vi "FightBot.vi"   [LabVIEW 2016, in "SumoRobot.lvrbt"]
uses:
  SumoRobot.lvrbt
  <vilib>/NXT/Block Support/NXT_OutputPort.ctl
  <vilib>/NXT/Block Support/NXT_InputPort.ctl
  <vilib>/NXT/Dual Mode Library/Sensors/Touch_Pressed.vi
  <vilib>/NXT/Dual Mode Library/Sensors/EV3_Color_Reflect.vi
  <vilib>/NXT/NXTIO Xnodes/NXTIONodeSubVIs/NXTMoveMotors.vi
  <vilib>/NXT/Dual Mode Library/Sensors/EV3_Ultrasonic_IN.vi
  <vilib>/NXT/Dual Mode Library/Display/drawNumber_float.vi
  <vilib>/NXT/Dual Mode Library/Display/drawText.vi
  <vilib>/NXT/Dual Mode Library/Sound/PlayRedPianoFile.vi
  <vilib>/NXT/Subs/LVHSConnector.ctl
  <vilib>/NXT/NXTIO Xnodes/AddressXNode/NXTIOAddress.xnode
  <vilib>/NXT/NXTIO Xnodes/NXTIOXNode/NXTIO.xnode
  <vilib>/NXT/LegoClasses/BrickReference/BrickReference.lvclass
types:
  T1 = typedef "NXT_InputPort.ctl" = u32
  T2 = typedef "NXT_OutputPort.ctl" = u8
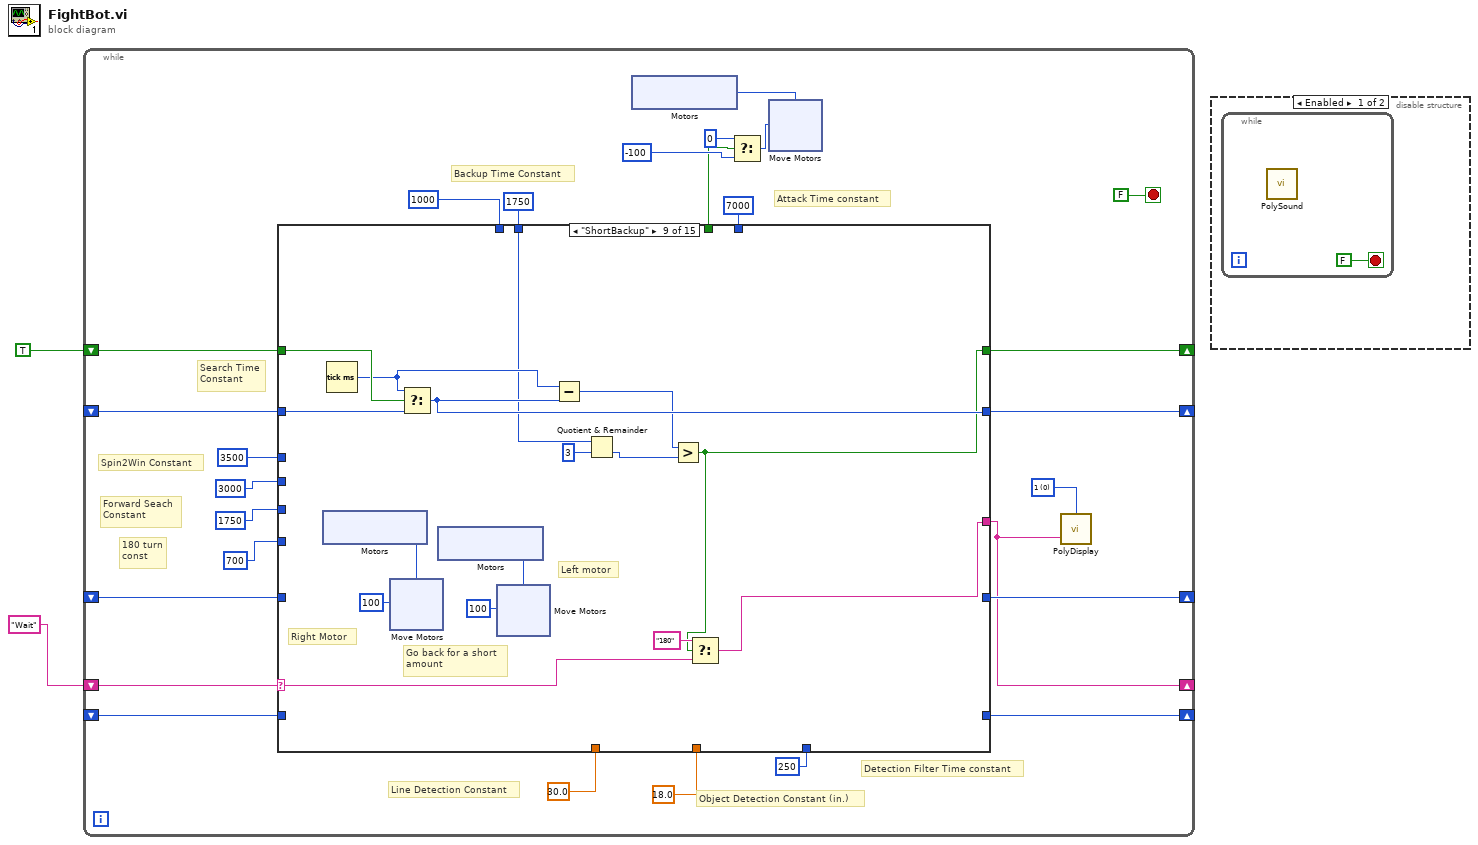
[diagram p0: block diagram]
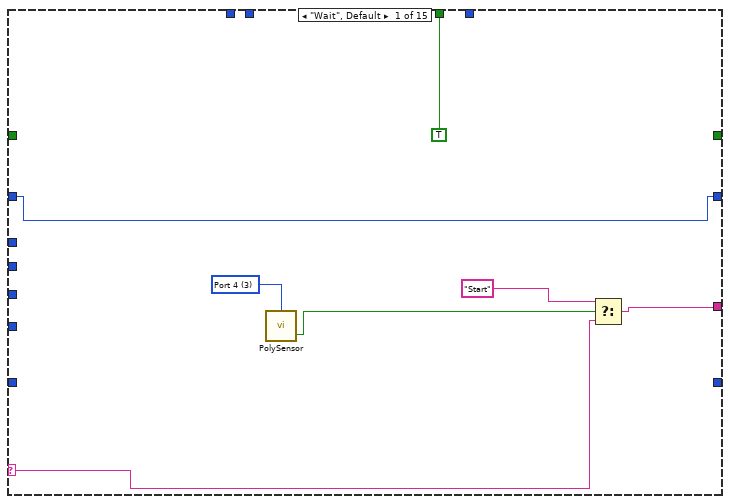
[diagram p3: hidden frame]
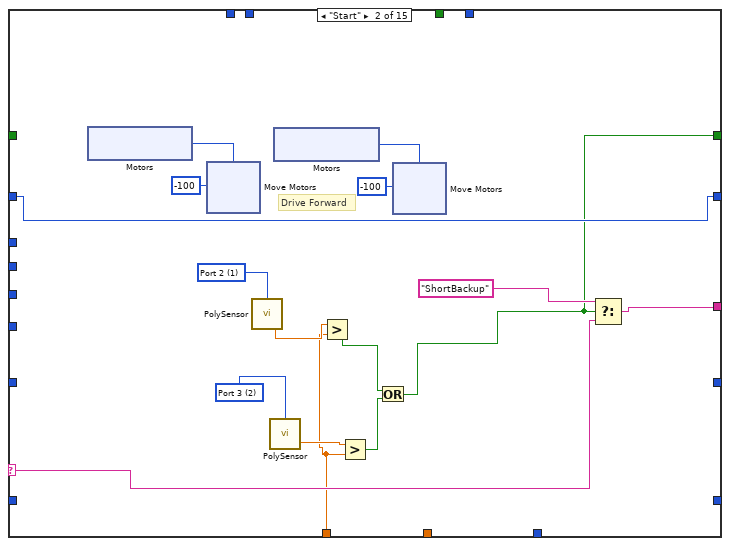
[diagram p4: hidden frame]
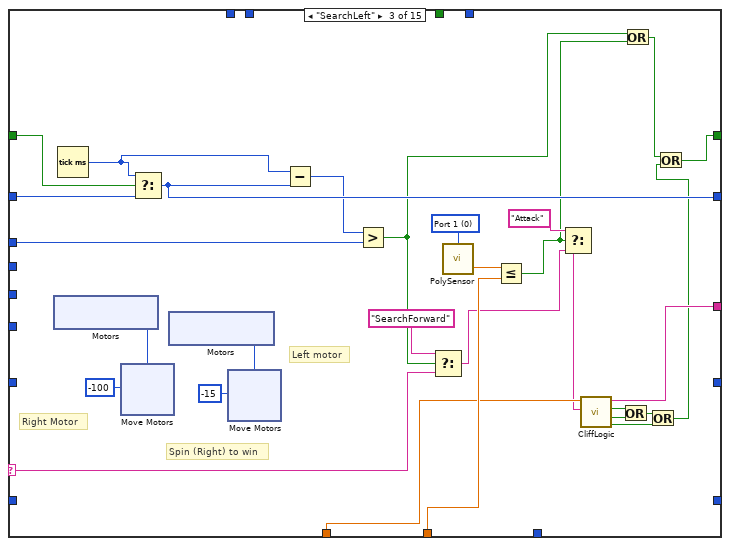
[diagram p5: hidden frame]
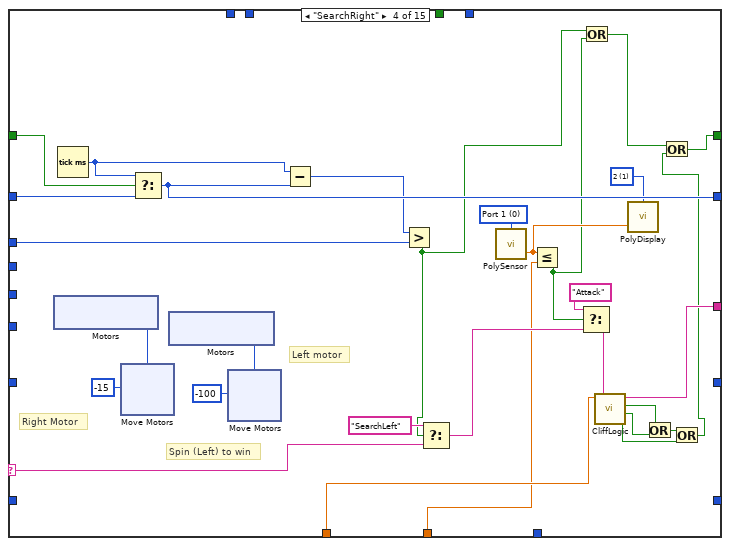
[diagram p6: hidden frame]
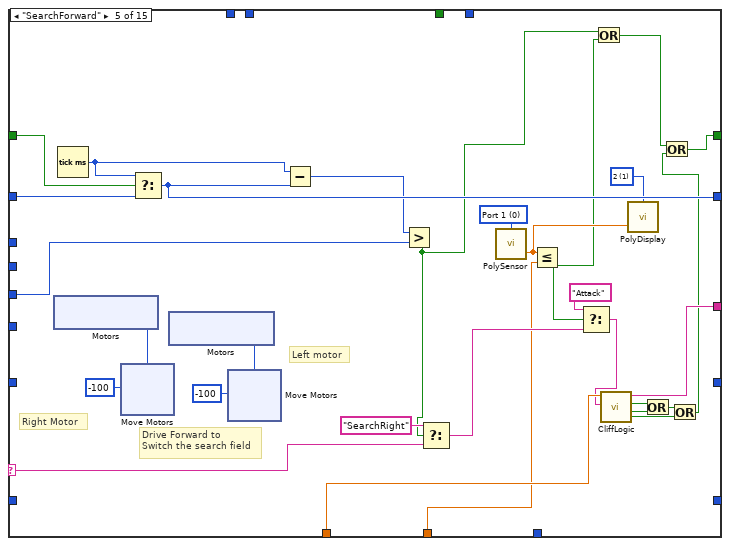
[diagram p7: hidden frame]
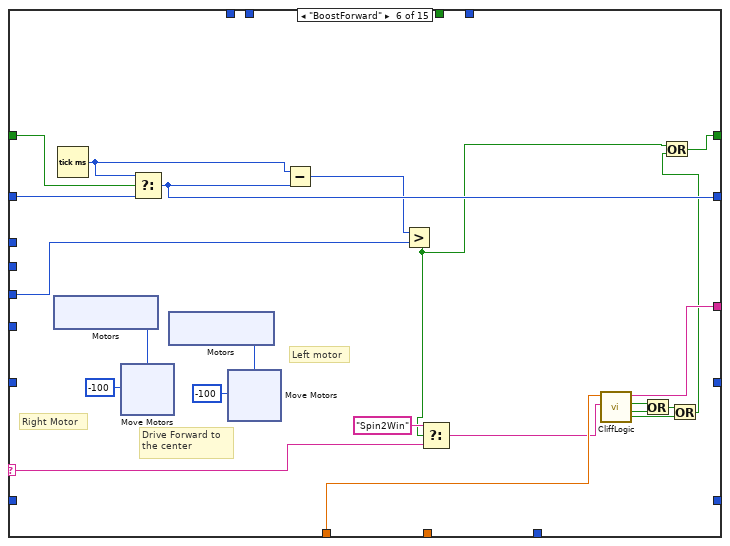
[diagram p8: hidden frame]
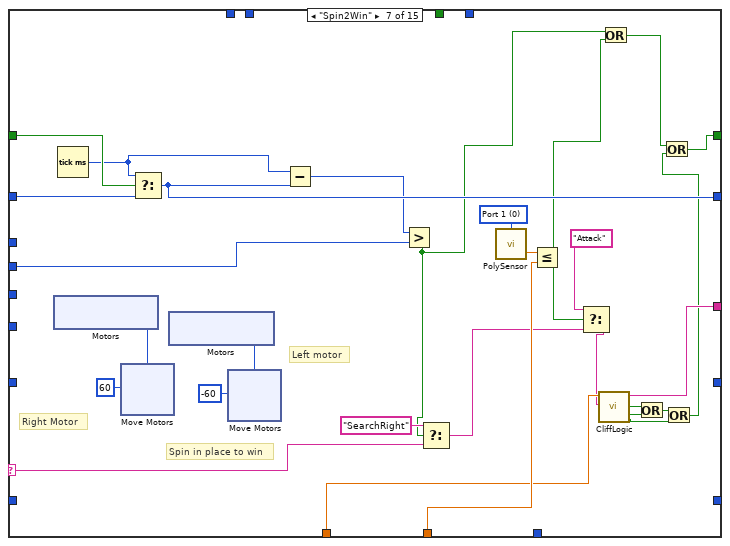
[diagram p9: hidden frame]
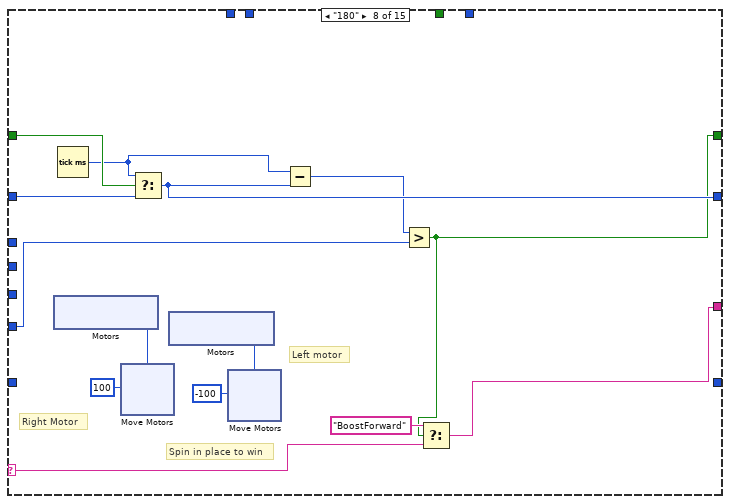
[diagram p10: hidden frame]
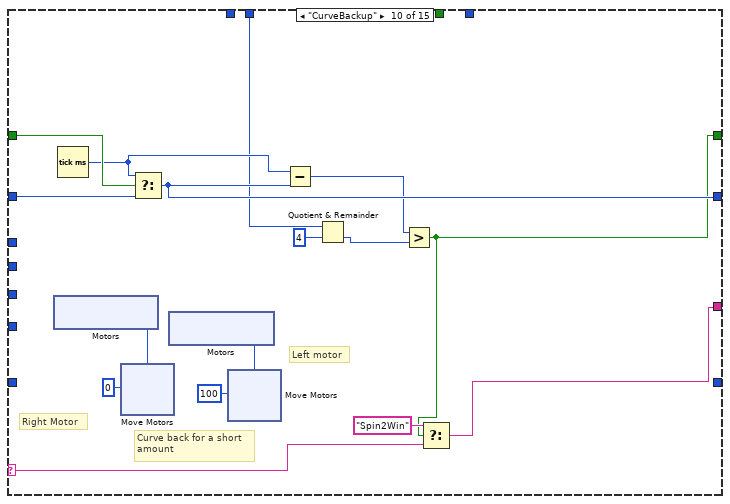
[diagram p11: hidden frame]
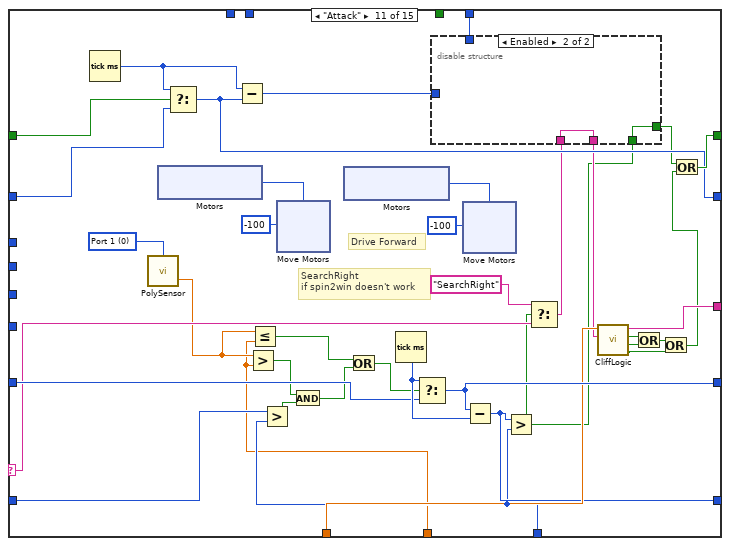
[diagram p12: hidden frame]
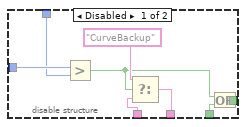
[diagram p13: hidden frame]
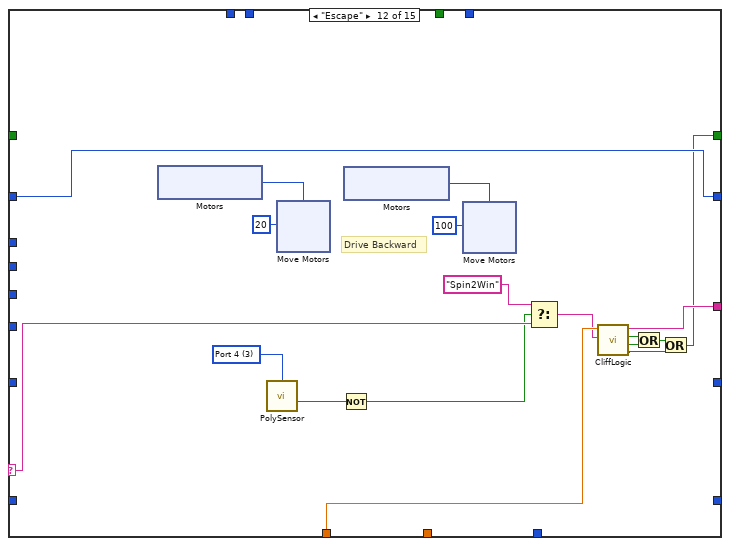
[diagram p14: hidden frame]
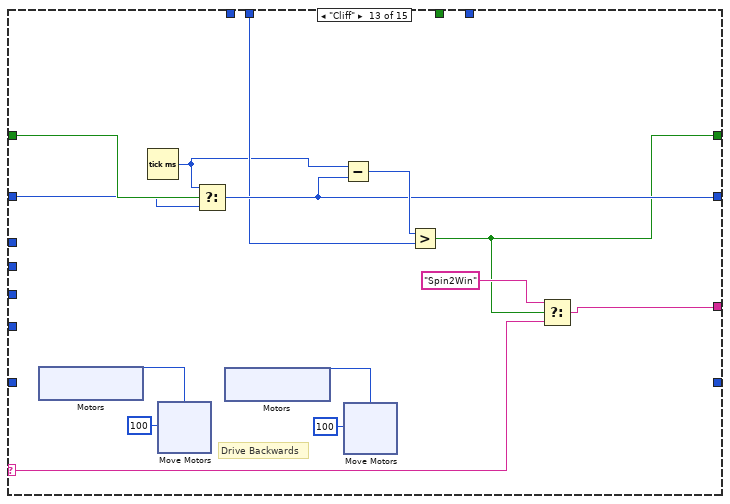
[diagram p15: hidden frame]
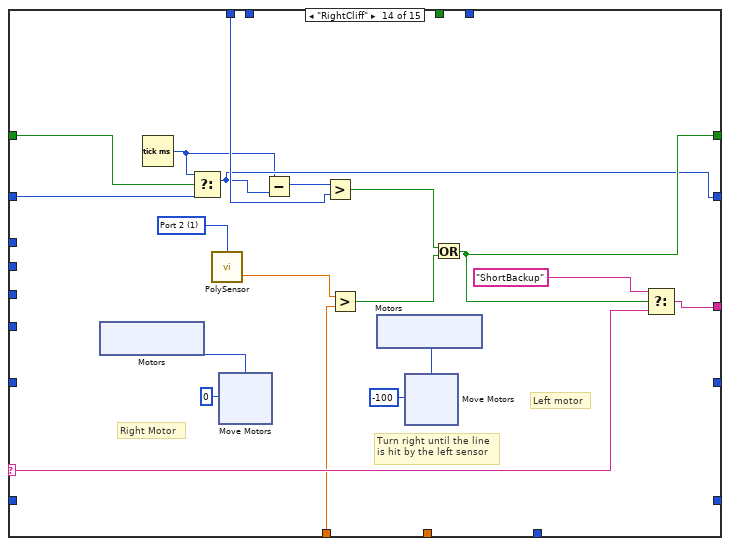
[diagram p16: hidden frame]
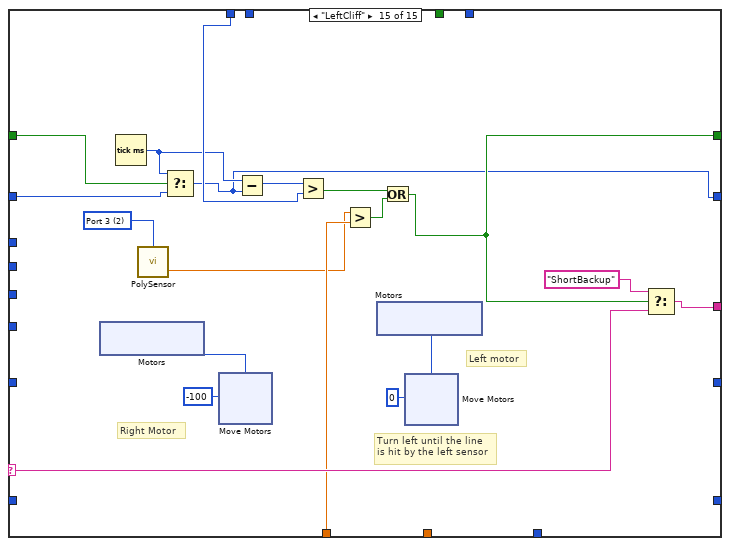
[diagram p17: hidden frame]
diagram:
  n1 = while {
    shift-right: [w13] -> _
    shift-left: "Wait" -> [w28]
    shift-right: [w25] -> _
    shift-left: TRUE -> [w24]
    shift-right: [w23] -> _
    shift-left: _ -> [w22]
    shift-right: [w18] -> _
    shift-left: _ -> [w17]
    shift-right: [w15] -> _
    shift-left: _ -> [w14]
    stop <- FALSE stop-if-true
    w12 = i16 0 items=["1", "2", "3", "4", "5", "6", "7", "8", "9", "10", "11", "12"] ("Line")
    # "Attack Time constant"
    # "180 turn\nconst"
    # "Forward Seach\nConstant"
    # "Spin2Win Constant"
    # "Detection Filter Time constant"
    # "Backup Time Constant"
    # "Search Time\nConstant"
    # "Object Detection Constant (in.)"
    # "Line Detection Constant"
    n2 = case shown="\"ShortBackup\"" w28 {
      selector: w28 -> [w43 w55 w90 w138 w185 w225 w266 w301 w333 w365 w419 w467 w501 w537 w572]
      tunnel: sgl 18.0 ("y") -> [_ _ w99 w133 w180 _ w274 _ _ _ w408 _ _ _ _]
      tunnel: sgl 30.0 ("y") -> [_ w46 w97 w145 w191 w231 w272 _ _ _ w418 w466 _ w529 w564]
      tunnel: [w42 w54 w87 w135 w182 w224 w263 w298 w331 w363 w417 w465 w490 w536 w571] -> w13
      tunnel: [_ w45 w86 w134 w181 w223 w262 w297 w330 w362 w416 w455 w492 w521 w556] -> w25
      tunnel: w24 -> [_ _ w96 w144 w190 w230 w271 w306 w338 w370 w399 _ w495 w527 w561]
      tunnel: [w41 w53 w94 w142 w188 w228 w269 w304 w336 w368 w398 w459 w493 w520 w554] -> w23
      tunnel: w22 -> [w41 w53 w95 w143 w189 w229 w270 w305 w337 w369 w400 w459 w494 w526 w559]
      tunnel: u32 3500 ("y") -> [_ _ w92 w140 _ _ _ _ _ _ _ _ _ _ _]
      tunnel: u32 1750 ("y") -> [_ _ _ _ _ _ _ _ w329 w361 _ _ w491 _ _]
      tunnel: u32 3000 ("y") -> [_ _ _ _ _ _ w261 _ _ _ _ _ _ _ _]
      tunnel: [_ _ _ _ _ _ _ _ _ _ w422 _ _ _ _] -> w18
      tunnel: w17 -> [_ _ _ _ _ _ _ _ _ _ w420 _ _ _ _]
      tunnel: u32 250 ("y") -> [_ _ _ _ _ _ _ _ _ _ w413 _ _ _ _]
      tunnel: [_ _ _ _ _ _ _ _ _ _ w415 _ _ _ _] -> w15
      tunnel: w14 -> [_ _ _ _ _ _ _ _ _ _ w414 _ _ _ _]
      tunnel: u32 1750 ("y") -> [_ _ _ _ w177 w222 _ _ _ _ _ _ _ _ _]
      tunnel: u32 700 ("y") -> [_ _ _ _ _ _ _ w299 _ _ _ _ _ _ _]
      tunnel: [TRUE _ _ _ _ _ _ _ _ _ _ _ _ _ _] -> w7
      tunnel: u32 1000 ("y") -> [_ _ _ _ _ _ _ _ _ _ _ _ _ w525 w560]
      tunnel: u32 7000 ("y") -> [_ _ _ _ _ _ _ _ _ _ w395 _ _ _ _]
      frame "Wait", Default {
        w39 = T1 3 items=["Port 1", "Port 2", "Port 3", "Port 4"] ("Port (Port 1)")
        n3 = call-poly <vilib>:"PolySensor.vi"("Port (Port 1)"=w39) -> ("Yes / No"=w40:bool)  [unwired: 2 in, 1 out]
        n4 = Select(t="Start", s=w40, f=w43) -> (s? t:f=w42:string)
      }
      frame "Start" {
        w49 = T1 2 items=["Port 1", "Port 2", "Port 3", "Port 4"] ("Port (Port 1)")
        w52 = T1 1 items=["Port 1", "Port 2", "Port 3", "Port 4"] ("Port (Port 1)")
        # "Drive Forward"
        n5 = xnode "Motors"() -> ("Motor"=w60:T2)
        n6 = xnode "Move Motors"("Power/Speed 1"=i8 -100, "Motors"=w60) -> ()  [unwired: 1 in, 1 out]
        n7 = call-poly <vilib>:"PolySensor.vi"("Port (Port 1)"=w52) -> ("Scaled Value"=w51:sgl)  [unwired: 2 in, 1 out]
        n8 = call-poly <vilib>:"PolySensor.vi"("Port (Port 1)"=w49) -> ("Scaled Value"=w50:sgl)  [unwired: 2 in, 1 out]
        n9 = xnode "Motors"() -> ("Motor"=w57:T2)
        n10 = Greater?(x=w51, y=w46) -> (0:w48:bool)
        n11 = Greater?(x=w50, y=w46) -> (0:w47:bool)
        n12 = Or(x=w48, y=w47) -> (x .or. y?=w45:bool)
        n13 = xnode "Move Motors"("Power/Speed 1"=i8 -100, "Motors"=w57) -> ()  [unwired: 1 in, 1 out]
        n14 = Select(t="ShortBackup", s=w45, f=w55) -> (s? t:f=w54:string)
      }
      frame "SearchLeft" {
        w101 = T1 0 items=["Port 1", "Port 2", "Port 3", "Port 4"] ("Port (Port 1)")
        # "Right Motor"
        # "Left motor"
        # "Spin (Right) to win"
        n15 = xnode "Motors"() -> ("Motor"=w105:T2)
        n16 = Tick Count (ms)() -> (millisecond timer value=w85:u32)
        n17 = xnode "Move Motors"("Power/Speed 1"=i8 -100, "Motors"=w105) -> ()  [unwired: 1 in, 1 out]
        n18 = Select(t=w85, s=w96, f=w95) -> (s? t:f=w94:u32)
        n19 = xnode "Motors"() -> ("Motor"=w102:T2)
        n20 = xnode "Move Motors"("Power/Speed 1"=i8 -15, "Motors"=w102) -> ()  [unwired: 1 in, 1 out]
        n21 = Subtract(x=w85, y=w94) -> (x-y=w93:u32)
        n22 = Greater?(x=w93, y=w92) -> (0:w78:bool)
        n23 = Select(t="SearchForward", s=w78, f=w90) -> (s? t:f=w89:string)
        n24 = call-poly <vilib>:"PolySensor.vi"("Port (Port 1)"=w101) -> ("Inches"=w100:sgl)  [unwired: 2 in, 1 out]
        n25 = Less Or Equal?(x=w100, y=w99) -> (x <= y?=w79:bool)
        n26 = Select(t="Attack", s=w79, f=w89) -> (s? t:f=w88:string)
        n27 = call "CliffLogic.vi"("State In"=w88, "Light Threshold"=w97) -> ("Both Light"=w81:bool, "Right Light"=w83:bool, "Left Light"=w84:bool, "State Out"=w87:string)  [unwired: 6 in]
        n28 = Or(x=w84, y=w83) -> (x .or. y?=w82:bool)
        n29 = Or(x=w78, y=w79) -> (x .or. y?=w77:bool)
        n30 = Or(x=w82, y=w81) -> (x .or. y?=w80:bool)
        n31 = Or(x=w77, y=w80) -> (x .or. y?=w86:bool)
      }
      frame "SearchRight" {
        w131 = i16 1 items=["1", "2", "3", "4", "5", "6", "7", "8", "9", "10", "11", "12"] ("Line")
        w147 = T1 0 items=["Port 1", "Port 2", "Port 3", "Port 4"] ("Port (Port 1)")
        # "Right Motor"
        # "Left motor"
        # "Spin (Left) to win"
        n32 = xnode "Motors"() -> ("Motor"=w151:T2)
        n33 = Tick Count (ms)() -> (millisecond timer value=w130:u32)
        n34 = xnode "Move Motors"("Power/Speed 1"=i8 -15, "Motors"=w151) -> ()  [unwired: 1 in, 1 out]
        n35 = Select(t=w130, s=w144, f=w143) -> (s? t:f=w142:u32)
        n36 = xnode "Motors"() -> ("Motor"=w148:T2)
        n37 = xnode "Move Motors"("Power/Speed 1"=i8 -100, "Motors"=w148) -> ()  [unwired: 1 in, 1 out]
        n38 = Subtract(x=w130, y=w142) -> (x-y=w141:u32)
        n39 = Greater?(x=w141, y=w140) -> (0:w123:bool)
        n40 = Select(t="SearchLeft", s=w123, f=w138) -> (s? t:f=w137:string)
        n41 = call-poly <vilib>:"PolySensor.vi"("Port (Port 1)"=w147) -> ("Inches"=w132:sgl)  [unwired: 2 in, 1 out]
        n42 = Less Or Equal?(x=w132, y=w133) -> (x <= y?=w124:bool)
        n43 = Select(t="Attack", s=w124, f=w137) -> (s? t:f=w136:string)
        n44 = Or(x=w123, y=w124) -> (x .or. y?=w122:bool)
        n45 = call "CliffLogic.vi"("State In"=w136, "Light Threshold"=w145) -> ("Both Light"=w128:bool, "Right Light"=w126:bool, "Left Light"=w127:bool, "State Out"=w135:string)  [unwired: 6 in]
        n46 = call-poly <vilib>:"PolyDisplay.vi"("number"=w132, "Line"=w131) -> ()  [unwired: 2 in, 1 out]
        n47 = Or(x=w127, y=w126) -> (x .or. y?=w129:bool)
        n48 = Or(x=w129, y=w128) -> (x .or. y?=w125:bool)
        n49 = Or(x=w122, y=w125) -> (x .or. y?=w134:bool)
      }
      frame "SearchForward" {
        w178 = i16 1 items=["1", "2", "3", "4", "5", "6", "7", "8", "9", "10", "11", "12"] ("Line")
        w193 = T1 0 items=["Port 1", "Port 2", "Port 3", "Port 4"] ("Port (Port 1)")
        # "Right Motor"
        # "Left motor"
        # "Drive Forward to \nSwitch the search field"
        n50 = xnode "Motors"() -> ("Motor"=w197:T2)
        n51 = Tick Count (ms)() -> (millisecond timer value=w176:u32)
        n52 = xnode "Move Motors"("Power/Speed 1"=i8 -100, "Motors"=w197) -> ()  [unwired: 1 in, 1 out]
        n53 = Select(t=w176, s=w190, f=w189) -> (s? t:f=w188:u32)
        n54 = xnode "Motors"() -> ("Motor"=w194:T2)
        n55 = xnode "Move Motors"("Power/Speed 1"=i8 -100, "Motors"=w194) -> ()  [unwired: 1 in, 1 out]
        n56 = Subtract(x=w176, y=w188) -> (x-y=w187:u32)
        n57 = Greater?(x=w187, y=w177) -> (0:w170:bool)
        n58 = Select(t="SearchRight", s=w170, f=w185) -> (s? t:f=w184:string)
        n59 = call-poly <vilib>:"PolySensor.vi"("Port (Port 1)"=w193) -> ("Inches"=w179:sgl)  [unwired: 2 in, 1 out]
        n60 = Less Or Equal?(x=w179, y=w180) -> (x <= y?=w169:bool)
        n61 = Select(t="Attack", s=w169, f=w184) -> (s? t:f=w183:string)
        n62 = Or(x=w170, y=w169) -> (x .or. y?=w168:bool)
        n63 = call "CliffLogic.vi"("State In"=w183, "Light Threshold"=w191) -> ("Both Light"=w172:bool, "Right Light"=w173:bool, "Left Light"=w174:bool, "State Out"=w182:string)  [unwired: 6 in]
        n64 = call-poly <vilib>:"PolyDisplay.vi"("number"=w179, "Line"=w178) -> ()  [unwired: 2 in, 1 out]
        n65 = Or(x=w174, y=w173) -> (x .or. y?=w175:bool)
        n66 = Or(x=w175, y=w172) -> (x .or. y?=w171:bool)
        n67 = Or(x=w168, y=w171) -> (x .or. y?=w181:bool)
      }
      frame "BoostForward" {
        # "Right Motor"
        # "Left motor"
        # "Drive Forward to \nthe center"
        n68 = xnode "Motors"() -> ("Motor"=w235:T2)
        n69 = Tick Count (ms)() -> (millisecond timer value=w221:u32)
        n70 = xnode "Move Motors"("Power/Speed 1"=i8 -100, "Motors"=w235) -> ()  [unwired: 1 in, 1 out]
        n71 = Select(t=w221, s=w230, f=w229) -> (s? t:f=w228:u32)
        n72 = xnode "Motors"() -> ("Motor"=w232:T2)
        n73 = xnode "Move Motors"("Power/Speed 1"=i8 -100, "Motors"=w232) -> ()  [unwired: 1 in, 1 out]
        n74 = Subtract(x=w221, y=w228) -> (x-y=w227:u32)
        n75 = Greater?(x=w227, y=w222) -> (0:w215:bool)
        n76 = Select(t="Spin2Win", s=w215, f=w225) -> (s? t:f=w214:string)
        n77 = call "CliffLogic.vi"("State In"=w214, "Light Threshold"=w231) -> ("Both Light"=w217:bool, "Right Light"=w218:bool, "Left Light"=w219:bool, "State Out"=w224:string)  [unwired: 6 in]
        n78 = Or(x=w219, y=w218) -> (x .or. y?=w220:bool)
        n79 = Or(x=w220, y=w217) -> (x .or. y?=w216:bool)
        n80 = Or(x=w215, y=w216) -> (x .or. y?=w223:bool)
      }
      frame "Spin2Win" {
        w276 = T1 0 items=["Port 1", "Port 2", "Port 3", "Port 4"] ("Port (Port 1)")
        # "Right Motor"
        # "Left motor"
        # "Spin in place to win"
        n81 = xnode "Motors"() -> ("Motor"=w280:T2)
        n82 = Tick Count (ms)() -> (millisecond timer value=w260:u32)
        n83 = xnode "Move Motors"("Power/Speed 1"=i8 60, "Motors"=w280) -> ()  [unwired: 1 in, 1 out]
        n84 = Select(t=w260, s=w271, f=w270) -> (s? t:f=w269:u32)
        n85 = xnode "Motors"() -> ("Motor"=w277:T2)
        n86 = xnode "Move Motors"("Power/Speed 1"=i8 -60, "Motors"=w277) -> ()  [unwired: 1 in, 1 out]
        n87 = Subtract(x=w260, y=w269) -> (x-y=w268:u32)
        n88 = Greater?(x=w268, y=w261) -> (0:w254:bool)
        n89 = Select(t="SearchRight", s=w254, f=w266) -> (s? t:f=w265:string)
        n90 = call-poly <vilib>:"PolySensor.vi"("Port (Port 1)"=w276) -> ("Inches"=w275:sgl)  [unwired: 2 in, 1 out]
        n91 = Less Or Equal?(x=w275, y=w274) -> (x <= y?=w253:bool)
        n92 = Select(t="Attack", s=w253, f=w265) -> (s? t:f=w264:string)
        n93 = call "CliffLogic.vi"("State In"=w264, "Light Threshold"=w272) -> ("Both Light"=w258:bool, "Right Light"=w257:bool, "Left Light"=w256:bool, "State Out"=w263:string)  [unwired: 6 in]
        n94 = Or(x=w254, y=w253) -> (x .or. y?=w252:bool)
        n95 = Or(x=w256, y=w257) -> (x .or. y?=w259:bool)
        n96 = Or(x=w259, y=w258) -> (x .or. y?=w255:bool)
        n97 = Or(x=w252, y=w255) -> (x .or. y?=w262:bool)
      }
      frame "180" {
        # "Right Motor"
        # "Left motor"
        # "Spin in place to win"
        n98 = xnode "Motors"() -> ("Motor"=w310:T2)
        n99 = Tick Count (ms)() -> (millisecond timer value=w300:u32)
        n100 = xnode "Move Motors"("Power/Speed 1"=i8 100, "Motors"=w310) -> ()  [unwired: 1 in, 1 out]
        n101 = Select(t=w300, s=w306, f=w305) -> (s? t:f=w304:u32)
        n102 = xnode "Motors"() -> ("Motor"=w307:T2)
        n103 = xnode "Move Motors"("Power/Speed 1"=i8 -100, "Motors"=w307) -> ()  [unwired: 1 in, 1 out]
        n104 = Subtract(x=w300, y=w304) -> (x-y=w303:u32)
        n105 = Greater?(x=w303, y=w299) -> (0:w297:bool)
        n106 = Select(t="BoostForward", s=w297, f=w301) -> (s? t:f=w298:string)
      }
      frame "ShortBackup" {
        # "Right Motor"
        # "Left motor"
        # "Go back for a short\namount"
        n107 = xnode "Motors"() -> ("Motor"=w342:T2)
        n108 = Tick Count (ms)() -> (millisecond timer value=w332:u32)
        n109 = xnode "Move Motors"("Power/Speed 1"=i8 100, "Motors"=w342) -> ()  [unwired: 1 in, 1 out]
        n110 = Select(t=w332, s=w338, f=w337) -> (s? t:f=w336:u32)
        n111 = xnode "Motors"() -> ("Motor"=w339:T2)
        n112 = xnode "Move Motors"("Power/Speed 1"=i8 100, "Motors"=w339) -> ()  [unwired: 1 in, 1 out]
        n113 = Subtract(x=w332, y=w336) -> (x-y=w335:u32)
        n114 = Quotient & Remainder(x=w329, y=u32 3) -> (floor(x/y)=w328:u32)  [unwired: 1 out]
        n115 = Greater?(x=w335, y=w328) -> (0:w330:bool)
        n116 = Select(t="180", s=w330, f=w333) -> (s? t:f=w331:string)
      }
      frame "CurveBackup" {
        # "Right Motor"
        # "Left motor"
        # "Curve back for a short\namount"
        n117 = xnode "Motors"() -> ("Motor"=w374:T2)
        n118 = Tick Count (ms)() -> (millisecond timer value=w364:u32)
        n119 = xnode "Move Motors"("Power/Speed 1"=i8 0, "Motors"=w374) -> ()  [unwired: 1 in, 1 out]
        n120 = Select(t=w364, s=w370, f=w369) -> (s? t:f=w368:u32)
        n121 = xnode "Motors"() -> ("Motor"=w371:T2)
        n122 = xnode "Move Motors"("Power/Speed 1"=i8 100, "Motors"=w371) -> ()  [unwired: 1 in, 1 out]
        n123 = Subtract(x=w364, y=w368) -> (x-y=w367:u32)
        n124 = Quotient & Remainder(x=w361, y=u32 4) -> (floor(x/y)=w360:u32)  [unwired: 1 out]
        n125 = Greater?(x=w367, y=w360) -> (0:w362:bool)
        n126 = Select(t="Spin2Win", s=w362, f=w365) -> (s? t:f=w363:string)
      }
      frame "Attack" {
        w424 = T1 0 items=["Port 1", "Port 2", "Port 3", "Port 4"] ("Port (Port 1)")
        # "SearchRight\nif spin2win doesn't work"
        # "Drive Forward"
        n127 = Tick Count (ms)() -> (millisecond timer value=w397:u32)
        n128 = call-poly <vilib>:"PolySensor.vi"("Port (Port 1)"=w424) -> ("Inches"=w409:sgl)  [unwired: 2 in, 1 out]
        n129 = xnode "Motors"() -> ("Motor"=w428:T2)
        n130 = Select(t=w397, s=w399, f=w400) -> (s? t:f=w398:u32)
        n131 = Subtract(x=w397, y=w398) -> (x-y=w396:u32)
        n132 = Greater?(x=w409, y=w408) -> (0:w411:bool)
        n133 = Less Or Equal?(x=w409, y=w408) -> (x <= y?=w407:bool)
        n134 = Greater?(x=w414, y=w413) -> (0:w412:bool)
        n135 = xnode "Move Motors"("Power/Speed 1"=i8 -100, "Motors"=w428) -> ()  [unwired: 1 in, 1 out]
        n136 = And(x=w411, y=w412) -> (x .and. y?=w410:bool)
        n137 = xnode "Motors"() -> ("Motor"=w425:T2)
        n138 = Or(x=w407, y=w410) -> (x .or. y?=w406:bool)
        n139 = Tick Count (ms)() -> (millisecond timer value=w421:u32)
        n140 = Select(t=w421, s=w406, f=w420) -> (s? t:f=w422:u32)
        n141 = xnode "Move Motors"("Power/Speed 1"=i8 -100, "Motors"=w425) -> ()  [unwired: 1 in, 1 out]
        n142 = Subtract(x=w422, y=w421) -> (x-y=w415:u32)
        n143 = Greater?(x=w415, y=w413) -> (0:w392:bool)
        n144 = Select(t="SearchRight", s=w392, f=w419) -> (s? t:f=w394:string)
        n145 = disable-structure shown="Enabled" {
          disable-tunnel: w396 -> [w436 _]
          disable-tunnel: w395 -> [w435 _]
          disable-tunnel: w394 -> [w434 w438]
          disable-tunnel: [w433 w438] -> w393
          disable-tunnel: w392 -> [w431 w437]
          disable-tunnel: [w429 w437] -> w391
          frame Disabled {
            n146 = Greater?(x=w436, y=w435) -> (0:w430:bool)
            n147 = Select(t="CurveBackup", s=w430, f=w434) -> (s? t:f=w433:string)
            n148 = Or(x=w430, y=w431) -> (x .or. y?=w429:bool)
          }
          frame Enabled {
          }
        }
        n149 = call "CliffLogic.vi"("State In"=w393, "Light Threshold"=w418) -> ("Both Light"=w402:bool, "Right Light"=w403:bool, "Left Light"=w404:bool, "State Out"=w417:string)  [unwired: 6 in]
        n150 = Or(x=w404, y=w403) -> (x .or. y?=w405:bool)
        n151 = Or(x=w405, y=w402) -> (x .or. y?=w401:bool)
        n152 = Or(x=w391, y=w401) -> (x .or. y?=w416:bool)
      }
      frame "Escape" {
        w458 = T1 3 items=["Port 1", "Port 2", "Port 3", "Port 4"] ("Port (Port 1)")
        # "Drive Backward"
        n153 = xnode "Motors"() -> ("Motor"=w472:T2)
        n154 = call-poly <vilib>:"PolySensor.vi"("Port (Port 1)"=w458) -> ("Yes / No"=w457:bool)  [unwired: 2 in, 1 out]
        n155 = xnode "Move Motors"("Power/Speed 1"=i8 20, "Motors"=w472) -> ()  [unwired: 1 in, 1 out]
        n156 = Not(x=w457) -> (.not. x?=w456:bool)
        n157 = xnode "Motors"() -> ("Motor"=w469:T2)
        n158 = xnode "Move Motors"("Power/Speed 1"=i8 100, "Motors"=w469) -> ()  [unwired: 1 in, 1 out]
        n159 = Select(t="Spin2Win", s=w456, f=w467) -> (s? t:f=w460:string)
        n160 = call "CliffLogic.vi"("State In"=w460, "Light Threshold"=w466) -> ("Both Light"=w461:bool, "Right Light"=w462:bool, "Left Light"=w463:bool, "State Out"=w465:string)  [unwired: 6 in]
        n161 = Or(x=w463, y=w462) -> (x .or. y?=w464:bool)
        n162 = Or(x=w464, y=w461) -> (x .or. y?=w455:bool)
      }
      frame "Cliff" {
        # "Drive Backwards"
        n163 = xnode "Motors"() -> ("Motor"=w499:T2)
        n164 = Tick Count (ms)() -> (millisecond timer value=w489:u32)
        n165 = xnode "Move Motors"("Power/Speed 1"=i8 100, "Motors"=w499) -> ()  [unwired: 1 in, 1 out]
        n166 = Select(t=w489, s=w495, f=w494) -> (s? t:f=w493:u32)
        n167 = xnode "Motors"() -> ("Motor"=w496:T2)
        n168 = Subtract(x=w489, y=w493) -> (x-y=w502:u32)
        n169 = xnode "Move Motors"("Power/Speed 1"=i8 100, "Motors"=w496) -> ()  [unwired: 1 in, 1 out]
        n170 = Greater?(x=w502, y=w491) -> (0:w492:bool)
        n171 = Select(t="Spin2Win", s=w492, f=w501) -> (s? t:f=w490:string)
      }
      frame "RightCliff" {
        w530 = T1 1 items=["Port 1", "Port 2", "Port 3", "Port 4"] ("Port (Port 1)")
        # "Right Motor"
        # "Left motor"
        # "Turn right until the line\nis hit by the left sensor"
        n172 = xnode "Motors"() -> ("Motor"=w534:T2)
        n173 = Tick Count (ms)() -> (millisecond timer value=w519:u32)
        n174 = Select(t=w519, s=w527, f=w526) -> (s? t:f=w520:u32)
        n175 = call-poly <vilib>:"PolySensor.vi"("Port (Port 1)"=w530) -> ("Scaled Value"=w528:sgl)  [unwired: 2 in, 1 out]
        n176 = xnode "Move Motors"("Power/Speed 1"=i8 0, "Motors"=w534) -> ()  [unwired: 1 in, 1 out]
        n177 = Subtract(x=w519, y=w520) -> (x-y=w524:u32)
        n178 = Greater?(x=w524, y=w525) -> (0:w523:bool)
        n179 = Greater?(x=w528, y=w529) -> (0:w522:bool)
        n180 = xnode "Motors"() -> ("Motor"=w531:T2)
        n181 = xnode "Move Motors"("Power/Speed 1"=i8 -100, "Motors"=w531) -> ()  [unwired: 1 in, 1 out]
        n182 = Or(x=w523, y=w522) -> (x .or. y?=w521:bool)
        n183 = Select(t="ShortBackup", s=w521, f=w537) -> (s? t:f=w536:string)
      }
      frame "LeftCliff" {
        w565 = T1 2 items=["Port 1", "Port 2", "Port 3", "Port 4"] ("Port (Port 1)")
        # "Right Motor"
        # "Left motor"
        # "Turn left until the line\nis hit by the left sensor"
        n184 = xnode "Motors"() -> ("Motor"=w569:T2)
        n185 = Tick Count (ms)() -> (millisecond timer value=w555:u32)
        n186 = call-poly <vilib>:"PolySensor.vi"("Port (Port 1)"=w565) -> ("Scaled Value"=w563:sgl)  [unwired: 2 in, 1 out]
        n187 = Select(t=w555, s=w561, f=w559) -> (s? t:f=w554:u32)
        n188 = xnode "Move Motors"("Power/Speed 1"=i8 -100, "Motors"=w569) -> ()  [unwired: 1 in, 1 out]
        n189 = Subtract(x=w555, y=w554) -> (x-y=w562:u32)
        n190 = Greater?(x=w562, y=w560) -> (0:w557:bool)
        n191 = Greater?(x=w563, y=w564) -> (0:w558:bool)
        n192 = xnode "Motors"() -> ("Motor"=w566:T2)
        n193 = Or(x=w557, y=w558) -> (x .or. y?=w556:bool)
        n194 = xnode "Move Motors"("Power/Speed 1"=i8 0, "Motors"=w566) -> ()  [unwired: 1 in, 1 out]
        n195 = Select(t="ShortBackup", s=w556, f=w572) -> (s? t:f=w571:string)
      }
    }
    n196 = xnode "Motors"() -> ("Motor"=w9:T2)
    n197 = Select(t=i8 0, s=w7, f=i8 -100 ("Power/Speed 1")) -> (s? t:f=w5:i8)
    n198 = xnode "Move Motors"("Power/Speed 1"=w5, "Motors"=w9) -> ()  [unwired: 1 in, 1 out]
    n199 = call-poly <vilib>:"PolyDisplay.vi"("Text"=w13, "Line"=w12) -> ()  [unwired: 2 in, 1 out]
  }
  n200 = disable-structure shown="Enabled" {
    frame Enabled {
      n201 = while {
        stop <- FALSE stop-if-true
        n202 = call-poly <vilib>:"PolySound.vi"() -> ()  [unwired: 4 in, 1 out]
      }
    }
    frame Disabled {
    }
  }
